vi "Raw_Data_File_Start_text.vi"(1 "Header length":i32) -> (0 "Start String":string)   [LabVIEW 2010]
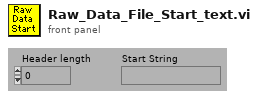
[diagram p1: front panel]
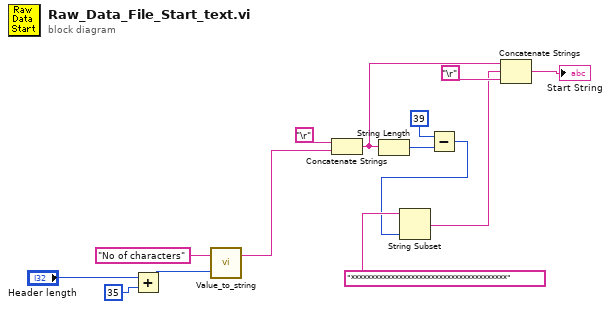
[diagram p0: block diagram]
diagram:
  n1 = Add(x="Header length", y=35) -> (x+y=w5:i32)
  n2 = call "Value_to_string.vi"("Value"=w5, "Label for value"="No of characters" ("Variable name")) -> ("Output string"=w3:string)  [unwired: 1 in]
  n3 = Concatenate Strings("\r", w3) -> (w11:string)
  n4 = String Length(string=w11) -> (length=w8:i32)
  n5 = Subtract(x=39 ("y"), y=w8) -> (x-y=w9:i32)
  n6 = String Subset(string="***************************************" ("Substring"), length (rest)=w9) -> (substring=w12:string)  [unwired: 1 out]
  n7 = Concatenate Strings(w11, w12, "\r") -> (→"Start String":string)
